vi "WriteFeaturesToMap.vi"(8 "error in (no error)":errorcluster, 10 "Map in":T6, 11 "Group":T1) -> (0 "error out":errorcluster, 2 "Map out":T6, 3 "Group out":T1)   [LabVIEW 2017, in "CmsAnalysis.lvlib"]
uses:
  <vilib>/addons/InsightCM/Devices/Shared/Cms/CmsAnalysis/CmsAnalysis.lvlib
  <vilib>/addons/PointValueMap/controls/PointMap.ctl
  <vilib>/addons/InsightCM/Devices/Shared/Cms/CmsAnalysis/controls/Group.ctl
  <vilib>/addons/InsightCM/Utilities/Analysis/Shared/controls/Channel.ctl
  <vilib>/addons/InsightCM/Utilities/Analysis/Shared/controls/SpeedType.ctl
  <vilib>/addons/InsightCM/Utilities/Analysis/Shared/controls/Feature.ctl
  <vilib>/addons/InsightCM/Utilities/Analysis/Shared/controls/AmplitudeScale.ctl
  <vilib>/addons/PointValueMap/subVIs/Point_Write_double.vi
  <vilib>/addons/PointValueMap/PointValueMap.lvlib
  <vilib>/addons/InsightCM/Utilities/Analysis/Shared/AnalysisHelper.lvlib
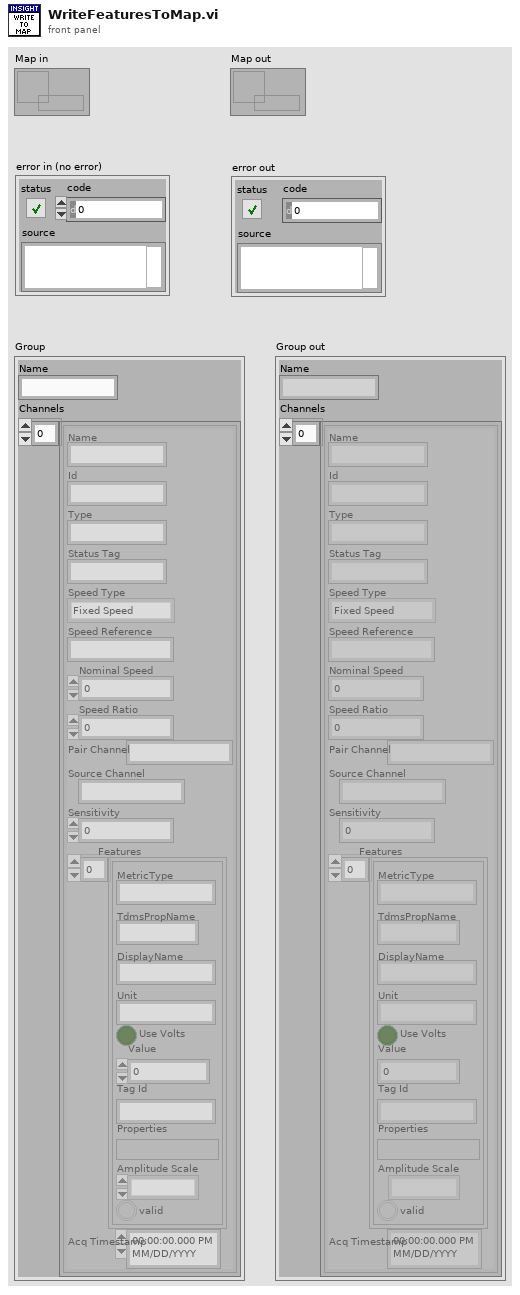
[diagram p1: front panel]
types:
  T1 = typedef "CmsAnalysis.lvlib/Group.ctl" = cluster{"Name":string, "Channels":T2[]}
  T2 = typedef "AnalysisHelper.lvlib/Channel.ctl" = cluster{"Name":string, "Id":string, "Type":string, "Status Tag":string, "Speed Type":T3, "Speed Reference":string, "Nominal Speed":dbl, "Speed Ratio":dbl, "Pair Channel":string, "Source Channel":string, "Sensitivity":dbl, "Features":T4[], "Acq Timestamp":timestamp}
  T3 = typedef "AnalysisHelper.lvlib/SpeedType.ctl" = enum16{"Fixed Speed", "Tachometer"}
  T4 = typedef "AnalysisHelper.lvlib/Feature.ctl" = cluster{"MetricType":string, "TdmsPropName":string, "DisplayName":string, "Unit":string, "Use Volts":bool, "Value":dbl, "Tag Id":string, "Properties":variant, "Amplitude Scale":T5, "valid":bool}
  T5 = typedef "AnalysisHelper.lvlib/AmplitudeScale.ctl" = enum16{"rms", "peak", "pk-pk"}
  T6 = typedef "PointValueMap.lvlib/PointMap.ctl" = refnum<data-value>
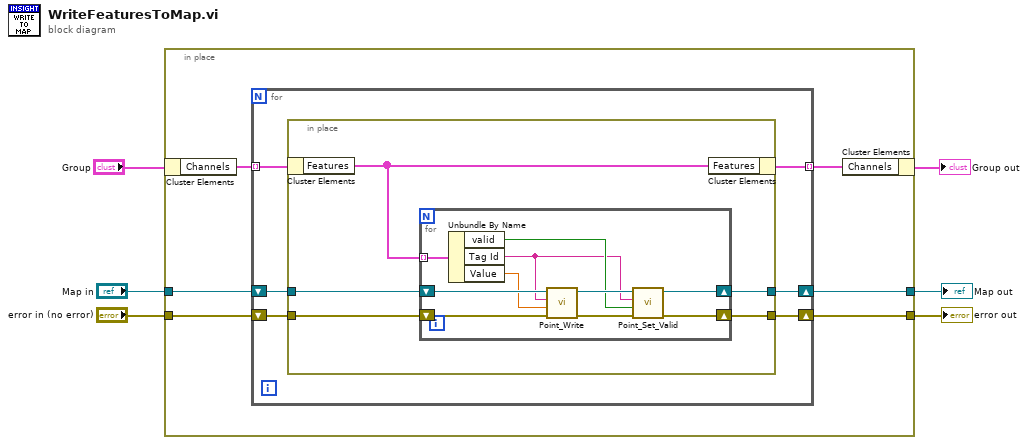
[diagram p0: block diagram]
diagram:
  n1 = in-place {
    in-place-border: "Map in" -> [w12]
    in-place-border: "error in (no error)" -> [w11]
    in-place-border: [w7] -> w6
    in-place-border: [w10] -> w3
    n2 = in-place-cluster #1("Group") -> ("Channels"=w9:T2[])
    n3 = for {
      tunnel: w9 -> [w18] mode=indexing
      shift-right: [w14] -> w10
      shift-left: w12 -> [w17]
      tunnel: [w13] -> w8 mode=indexing
      shift-right: [w15] -> w7
      shift-left: w11 -> [w16]
      n4 = in-place {
        in-place-border: w17 -> [w23]
        in-place-border: w16 -> [w22]
        in-place-border: [w19] -> w15
        in-place-border: [w21] -> w14
        n5 = in-place-cluster #2(w18) -> ("Features"=w20:T4[])
        n6 = for {
          tunnel: w20 -> [w33] mode=indexing
          shift-right: [w26] -> w21
          shift-left: w23 -> [w32]
          shift-right: [w28] -> w19
          shift-left: w22 -> [w31]
          n7 = Unbundle By Name(w33) -> ("valid"=w25:bool, "Tag Id"=w24:string, "Value"=w30:dbl)
          n8 = call-poly <vilib>:"Point_Write.vi"("Error In"=w31, "Value"=w30, "Tag"=w24, "Map"=w32) -> ("Error Out"=w29:errorcluster, "Map Out"=w27:T6)  [unwired: 6 in]
          n9 = call <vilib>:"Point_Set_Valid.vi"("Error In"=w29, "Valid?"=w25, "Tag"=w24, "Map"=w27) -> ("Error Out"=w28:errorcluster, "Map Out"=w26:T6)  [unwired: 6 in]
        }
        n10 = in-place-cluster #2("Features"=w20) -> (w13:T2)
      }
    }
    n11 = in-place-cluster #1("Channels"=w8) -> (→"Group out":T1)
  }
  "error out" <- w6
  "Map out" <- w3
